vi "randn_approximation.vi"(1 "normalize to +/-1 (True)":bool=TRUE, 2 "N":i32) -> (0 "randn() vector":dbl[](array[numeric]))   [LabVIEW 2013, in "dsdll.lvlib"]
doc: "Normal distribution random number generator (aproximation)."
uses:
  dsdll.lvlib
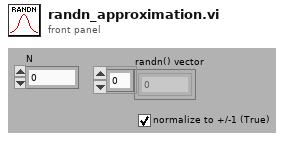
[diagram p1: front panel]
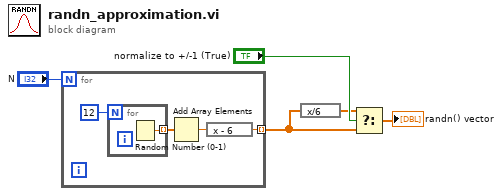
[diagram p0: block diagram]
diagram:
  n1 = for {
    N: "N" -> [_]
    tunnel: [w6] -> w1 mode=indexing
    n2 = for {
      N: 12 -> [_]
      tunnel: [w10] -> w8 mode=indexing
      n3 = Random Number (0-1)() -> (number: 0 to 1=w10:dbl)
    }
    n4 = Add Array Elements(numeric array=w8) -> (sum=w7:dbl)
    n5 = expression code="x - 6"(w7) -> (w6:dbl)
  }
  n6 = expression code="x/6"(w1) -> (w2:dbl[])
  n7 = Select(t=w2, s="normalize to +/-1 (True)", f=w1) -> (s? t:f=→"randn() vector":dbl[])
